vi "measureGraphsSD.vi"(0 "II channel seq":T2, 1 "OD averaged":dbl[](array[numeric]), 2 "Real Time Experiment":refnum<vi>, 3 "I channel seq":T2) -> ()   [LabVIEW 2015]
uses:
  controls/data-cluster.ctl
  globalVarSD.vi
panel:
  out "XY Graph":T1(graph)
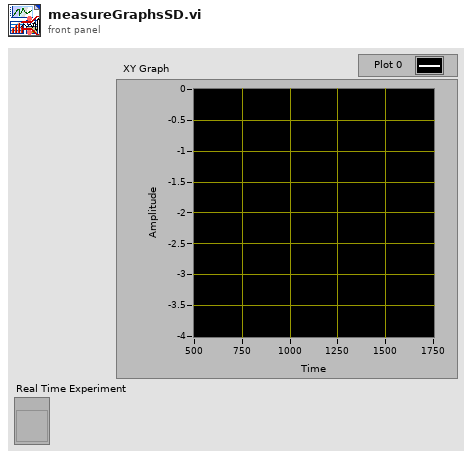
[diagram p1: front panel]
types:
  T1 = cluster{"wavelengths":dbl[], "OD averaged":dbl[]}[]
  T2 = typedef "data-cluster.ctl" = cluster{"BG":i32[], "Ie":i32[], "I0":i32[]}[]
  T3 = cluster{"wavelengths":dbl[], "OD averaged":dbl[]}
  T4 = cluster{"wavelengths":dbl[], "out array":dbl[]}[]
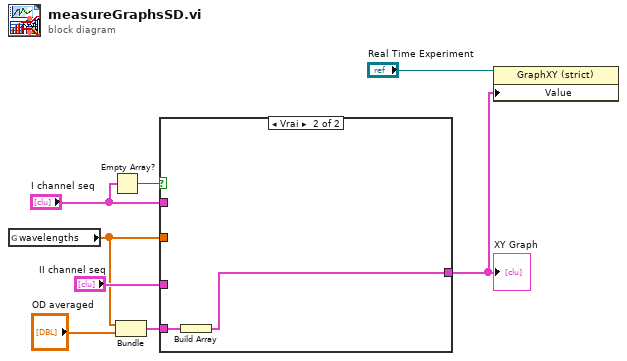
[diagram p0: block diagram]
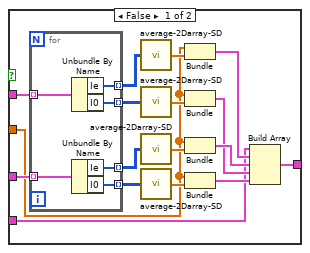
[diagram p2: hidden frame]
diagram:
  n1 = global read "globalVarSD.vi" "wavelengths"() -> (w5:dbl[])
  n2 = Empty Array?(array="I channel seq") -> (empty?=w3:bool)
  n3 = Bundle("wavelengths"=w5, "OD averaged"="OD averaged") -> (w7:T3)  [unwired: 1 in]
  n4 = case shown="Vrai" w3 {
    tunnel: [w21 w33] -> w2
    tunnel: w7 -> [w20 w32]
    tunnel: "I channel seq" -> [w19 _]
    tunnel: "II channel seq" -> [w18 _]
    tunnel: w5 -> [w9 _]
    frame False {
      n5 = for {
        tunnel: w19 -> [w31] mode=indexing
        tunnel: w18 -> [w30] mode=indexing
        tunnel: [w29] -> w17 mode=indexing
        tunnel: [w28] -> w16 mode=indexing
        tunnel: [w27] -> w15 mode=indexing
        tunnel: [w26] -> w14 mode=indexing
        n6 = Unbundle By Name(w31) -> ("Ie"=w29:i32[], "I0"=w28:i32[])
        n7 = Unbundle By Name(w30) -> ("Ie"=w27:i32[], "I0"=w26:i32[])
      }
      n8 = call "average-2Darray-SD.vi"("2D array"=w17) -> ("out array"=w13:dbl[])
      n9 = call "average-2Darray-SD.vi"("2D array"=w16) -> ("out array"=w12:dbl[])
      n10 = call "average-2Darray-SD.vi"("2D array"=w15) -> ("out array"=w11:dbl[])
      n11 = call "average-2Darray-SD.vi"("2D array"=w14) -> ("out array"=w10:dbl[])
      n12 = Bundle("wavelengths"=w9, "out array"=w13) -> (w25:cluster{"wavelengths":dbl[], "out array":dbl[]})  [unwired: 1 in]
      n13 = Bundle("wavelengths"=w9, "out array"=w12) -> (w23:cluster{"wavelengths":dbl[], "out array":dbl[]})  [unwired: 1 in]
      n14 = Bundle("wavelengths"=w9, "out array"=w11) -> (w24:cluster{"wavelengths":dbl[], "out array":dbl[]})  [unwired: 1 in]
      n15 = Bundle("wavelengths"=w9, "out array"=w10) -> (w22:cluster{"wavelengths":dbl[], "out array":dbl[]})  [unwired: 1 in]
      n16 = Build Array(w20, w25, w24, w23, w22) -> (w21:T4)
    }
    frame True {
      n17 = Build Array(w32) -> (w33:T1)
    }
  }
  "XY Graph" <- w2
  n18 = property class="GraphXY (strict)"(reference="Real Time Experiment", "Value"=w2) -> ()  [unwired: 1 in, 2 out]
